vi "调整表格列数_平均.vi"(8 "错误输入（无错误）":errorcluster, 10 "列数":i32, 11 "表格引用输入":refnum<vi>) -> (0 "错误输出":errorcluster, 3 "表格引用输出":refnum<vi>)   [LabVIEW 2014, in "表格.lvlib"]
uses:
  <vilib>/Utility/miscctls.llb/LVRowAndColumnTypeDef.ctl
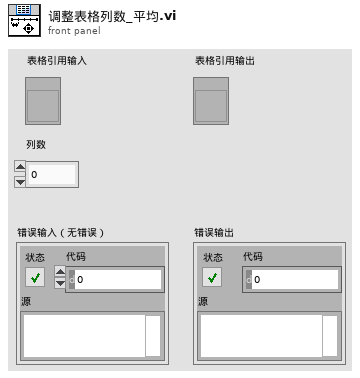
[diagram p1: front panel]
types:
  T1 = typedef "LVRowAndColumnTypeDef.ctl" = cluster{"Row":i32, "Column":i32}
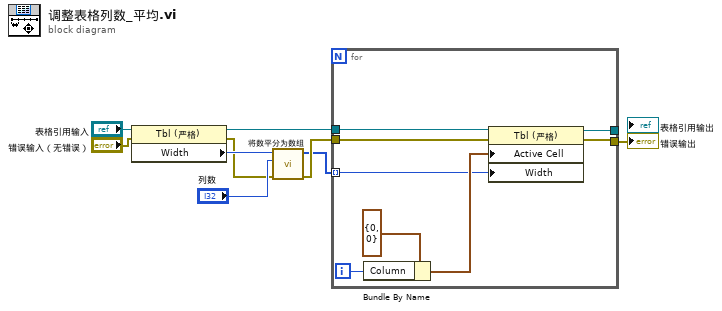
[diagram p0: block diagram]
diagram:
  n1 = property class="Tbl (严格)"(reference="表格引用输入", error in="错误输入（无错误）") -> (reference out=w9:refnum<vi>, error out=w3:errorcluster, "Width"=w7:u32)
  n2 = call "将数平分为数组.vi"("error in (no error)"=w3, "平分的分数"="列数", "数值"=w7) -> ("error out"=w5:errorcluster, "数组"=w1:u32[])  [unwired: 7 in]
  n3 = for {
    tunnel: w9 -> [w17]
    tunnel: w1 -> [w13] mode=indexing
    tunnel: w5 -> [w12]
    tunnel: [w11] -> w4
    tunnel: [w10] -> _
    i -> [w15]
    n4 = Bundle By Name(cluster=T1 {"Row"=0, "Column"=0} ("活动单元格:活动单元格"), "Column"=w15) -> (w14:T1)
    n5 = property class="Tbl (严格)"(reference=w17, error in=w12, "Active Cell"=w14, "Width"=w13) -> (reference out=w10:refnum<vi>, error out=w11:errorcluster)
  }
  "错误输出" <- w4
